vi "NI-Linux-RT Shared Library Path.vi"() -> (0 "Path":path)   [LabVIEW 2020, in "toolkit.lvlib"]
doc: "Obtain the path to the Shared Library on NI Linux RT"
uses:
  toolkit.lvlib
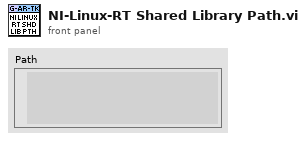
[diagram p1: front panel]
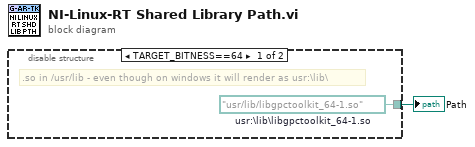
[diagram p0: block diagram]
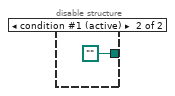
[diagram p2: hidden frame]
diagram:
  n1 = disable-structure shown="TARGET_BITNESS==64" {
    disable-tunnel: [w2 path ""] -> w1
    frame condition #0 {
      w2 = path "/usr/lib/libgpctoolkit_64-1.so"  # usr:\lib\libgpctoolkit_64-1.so
      # ".so in /usr/lib - even though on windows it will render as usr:\\lib\\"
    }
    frame condition #1 (active) {
    }
  }
  "Path" <- w1
